vi "pico_setup.vi"(8 "error in":errorcluster, 10 "PicoScope Acquisition Settings":T1={"Channel A Settings"={"Enabled"=TRUE, "Coupling"=1, "Range"=6, "Analogue Offset"=0.0}, "Channel B Settings"={"Enabled"=TRUE, "Coupling"=1, "Range"=6, "Analogue Offset"=0.0}, "Trigger Options"={"Trigger Enabled"=FALSE, "Trigger Source"=enum."Channel A", "Trigger Threshold (-5 to 5 V)"=0.0, "Trigger Slope"=2, "Trigger Delay (s)"=0.0, "Auto Trigger Time (ms)"=1000}, "Pico Scope Inititalization Settings"={"USB Power"=FALSE, "Use Serial Number"=FALSE, "Resolution"=0, "Serial Number"="", "Handle"=0}, "Use PicoScope?"=FALSE, "Acquisition Settings"={"Pre Trigger Time (s)"=512.0, "Post Trigger Time (s)"=512.0, "Resolution (s)"=36.0, "Four Channel Device"=FALSE, "Number of Captures"=1.0}} {"Acquisition Settings"."Number of Captures" min=1.0 step=1.0; "Acquisition Settings"."Resolution (s)" min=8e-09 max=36.0 step=8e-09 format="%.0p"; "Acquisition Settings"."Post Trigger Time (s)" min=0.0 format="%#_6p"; "Acquisition Settings"."Pre Trigger Time (s)" min=0.0 format="%#_6p"; "Pico Scope Inititalization Settings"."Resolution" items=["8-bit", "12-bit", "14-bit", "15-bit (max. 2 ch.)", "16-bit (max. 1 ch.)"]; "Trigger Options"."Trigger Slope" items=["Rising"=2, "Falling"=3]; "Channel B Settings"."Range" items=["10 mV", "20 mV", "50 mV", "100 mV", "200 mV", "500 mV", "1 V", "2 V", "5 V", "10 V", "20 V", "50 V ", "100 V"]; "Channel B Settings"."Coupling" items=["AC", "DC"]; "Channel A Settings"."Range" items=["10 mV", "20 mV", "50 mV", "100 mV", "200 mV", "500 mV", "1 V", "2 V", "5 V", "10 V", "20 V", "50 V ", "100 V"]; "Channel A Settings"."Coupling" items=["AC", "DC"]}, 11 "Call Num":i32) -> (0 "error out":errorcluster)   [LabVIEW 2016]
uses:
  Controls/PicoScope/pico_control_panel.ctl
  Controls/PicoScope/pico_channel_settings.ctl
  Controls/PicoScope/pico_trigger.ctl
  Controls/PicoScope/pico_init_settings.ctl
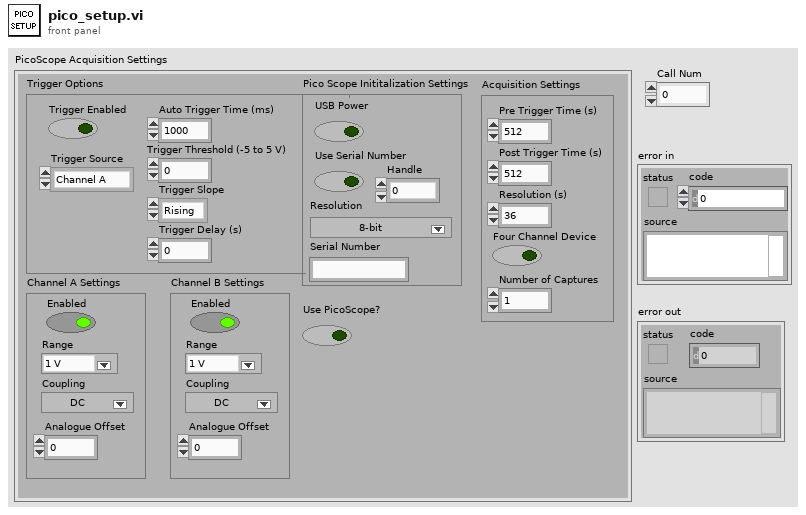
[diagram p1: front panel]
types:
  T1 = typedef "pico_control_panel.ctl" = cluster{"Channel A Settings":T2, "Channel B Settings":T2, "Trigger Options":T3, "Pico Scope Inititalization Settings":T4, "Use PicoScope?":bool, "Acquisition Settings":cluster{"Pre Trigger Time (s)":dbl, "Post Trigger Time (s)":dbl, "Resolution (s)":dbl, "Four Channel Device":bool, "Number of Captures":dbl}}
  T2 = typedef "pico_channel_settings.ctl" = cluster{"Enabled":bool, "Coupling":i16, "Range":u16, "Analogue Offset":sgl}
  T3 = typedef "pico_trigger.ctl" = cluster{"Trigger Enabled":bool, "Trigger Source":enum16{"Channel A", "Channel B", "Channel C", "Channel D", "Ext."}, "Trigger Threshold (-5 to 5 V)":dbl, "Trigger Slope":u16, "Trigger Delay (s)":dbl, "Auto Trigger Time (ms)":i16}
  T4 = typedef "pico_init_settings.ctl" = cluster{"USB Power":bool, "Use Serial Number":bool, "Resolution":i32, "Serial Number":string, "Handle":i16}
  T5 = cluster{"Trigger Enabled":bool, "Trigger Source":enum16{"Channel A", "Channel B", "Channel C", "Channel D", "Ext."}, "Trigger Threshold (16-bit counts)":i16, "Trigger Direction":u16, "Trigger Delay (samples)":u32, "Auto Trigger Time (ms)":i16}
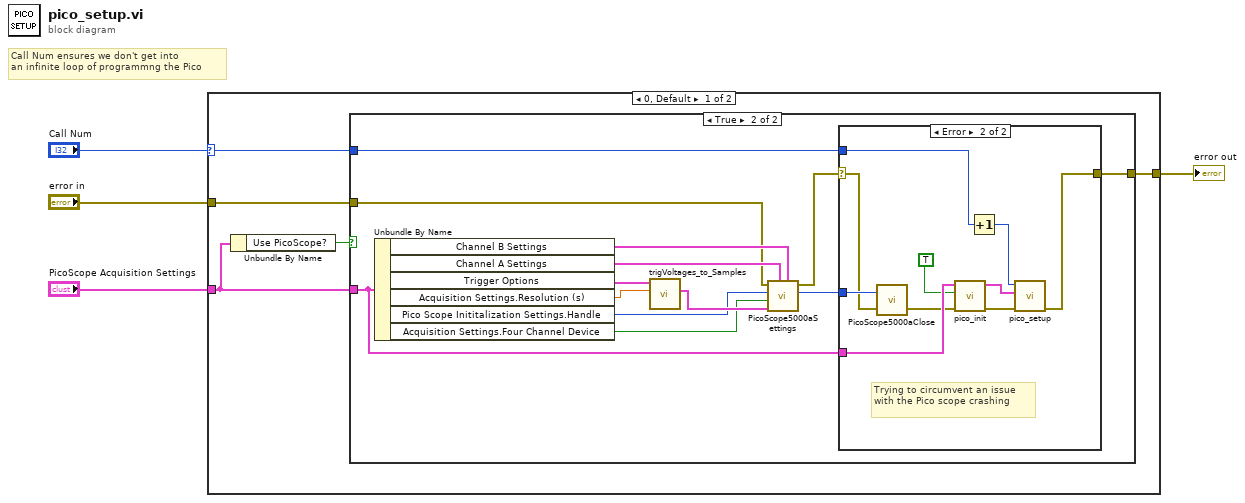
[diagram p0: block diagram]
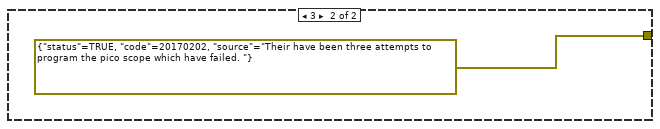
[diagram p4: hidden frame]
diagram:
  # "Call Num ensures we don't get into\nan infinite loop of programmng the Pico"
  n1 = case shown="0, Default" "Call Num" {
    selector: "Call Num" -> [w5 _]
    tunnel: "PicoScope Acquisition Settings" -> [w8 _]
    tunnel: "error in" -> [w7 _]
    tunnel: [w6 errorcluster {"status"=TRUE, "code"=20170202, "source"="Their have been three attempts to program the pico scope which have failed. "} ("error in")] -> w2
    frame 0, Default {
      n2 = Unbundle By Name(w8) -> ("Use PicoScope?"=w9:bool)
      n3 = case shown="True" w9 {
        tunnel: w8 -> [_ w12]
        tunnel: w7 -> [w10 w21]
        tunnel: [w10 w14] -> w6
        tunnel: w5 -> [_ w11]
        frame False {
        }
        frame True {
          n4 = Unbundle By Name(w12) -> ("Channel B Settings"=w22:T2, "Channel A Settings"=w23:T2, "Trigger Options"=w20:T3, "Acquisition Settings.Resolution (s)"=w19:dbl, "Pico Scope Inititalization Settings.Handle"=w16:i16, "Acquisition Settings.Four Channel Device"=w17:bool)
          n5 = call "trigVoltages_to_Samples.vi"("resolution (s)"=w19, "Trigger Options"=w20) -> ("Trigger Settings"=w18:T5)  [unwired: 9 in]
          n6 = call "PicoScope5000aSettings.vi"("Channel B Settings"=w22, "Channel A Settings"=w23, "Trigger Settings"=w18, "Four Channel Device?"=w17, "handle in"=w16, "error in"=w21) -> ("handle out"=w13:i16, "error out"=w15:errorcluster)  [unwired: 4 in]
          n7 = case shown="Error" w15 {
            selector: w15 -> [w24 w32]
            tunnel: [w24 w34] -> w14
            tunnel: w13 -> [_ w33]
            tunnel: w12 -> [_ w31]
            tunnel: w11 -> [_ w25]
            frame No Error {
            }
            frame Error {
              # "Trying to circumvent an issue with the Pico scope crashing"
              n8 = call "PicoScope5000aClose.vi"("error in (no error)"=w32, "handle"=w33) -> ("error out"=w30:errorcluster)  [unwired: 1 in]
              n9 = call "pico_init.vi"("error in (no error)"=w30, "Initialize PicoScope?"=TRUE, "PicoScope Acquisition Settings Input"=w31) -> ("error out"=w27:errorcluster, "PicoScope Acquisition Settings Output"=w28:T1)  [unwired: 4 in, 2 out]
              n10 = Increment(x=w25) -> (x+1=w26:i32)
              n11 = call "pico_setup.vi"("error in"=w27, "PicoScope Acquisition Settings"=w28, "Call Num"=w26) -> ("error out"=w34:errorcluster)  [unwired: 8 in]
            }
          }
        }
      }
    }
    frame 3 {
    }
  }
  "error out" <- w2
